vi "Parse Passport String.vi"(11 "Passport String":string) -> (0 "Why Bad":T1, 1 "Valid?":bool, 3 "Passport Info":T2)   [LabVIEW 2020]
uses:
  Typedefs/Passport.ctl
  Typedefs/ecl.ctl
  <vilib>/Utility/Data Type/NI_Data Type.lvlib
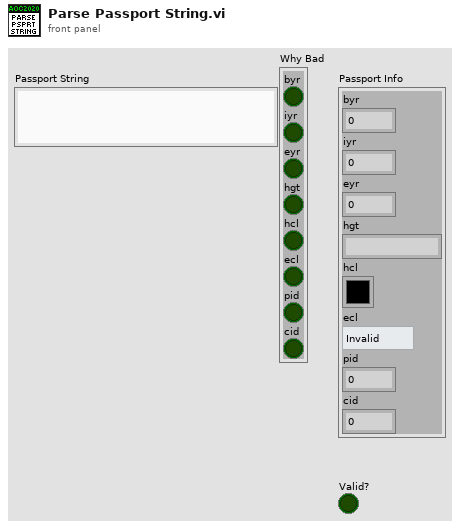
[diagram p1: front panel]
types:
  T1 = cluster{"byr":bool, "iyr":bool, "eyr":bool, "hgt":bool, "hcl":bool, "ecl":bool, "pid":bool, "cid":bool}
  T2 = typedef "Passport.ctl" = cluster{"byr":i32, "iyr":i32, "eyr":i32, "hgt":string, "hcl":u32, "ecl":T3, "pid":i32, "cid":i32}
  T3 = typedef "ecl.ctl" = enum16{"Invalid", "amb", "blu", "brn", "gry", "grn", "hzl", "oth"}
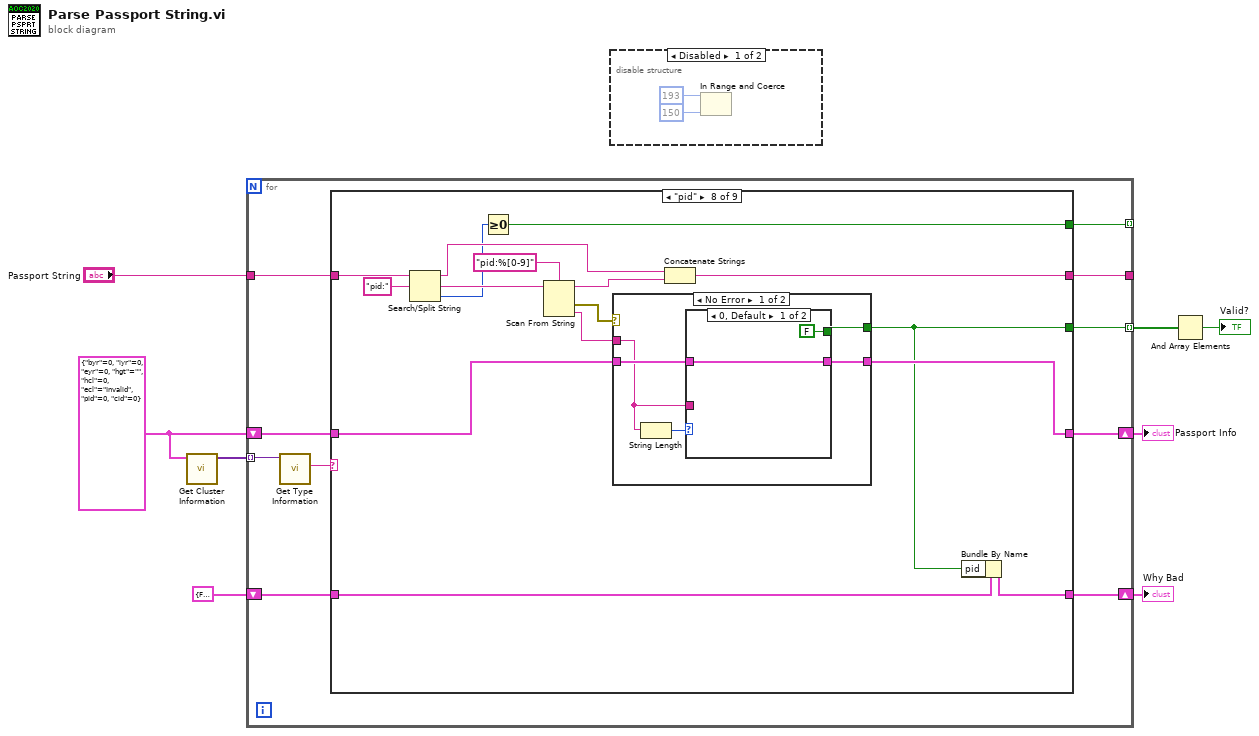
[diagram p0: block diagram]
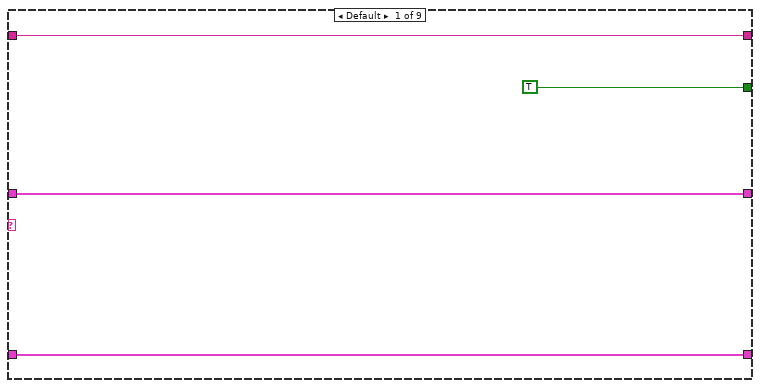
[diagram p3: hidden frame]
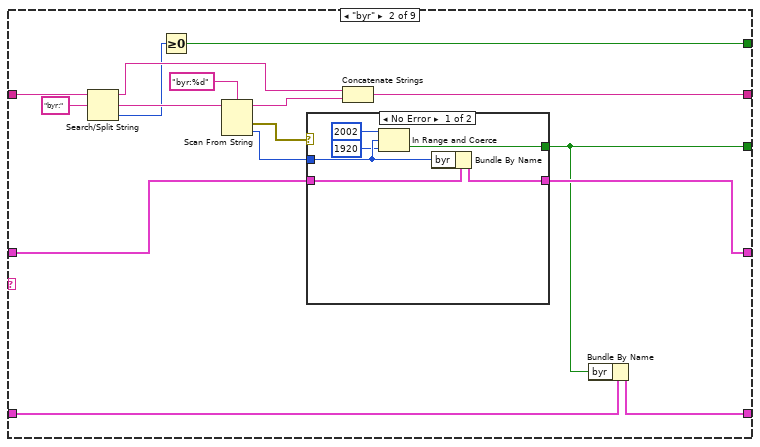
[diagram p4: hidden frame]
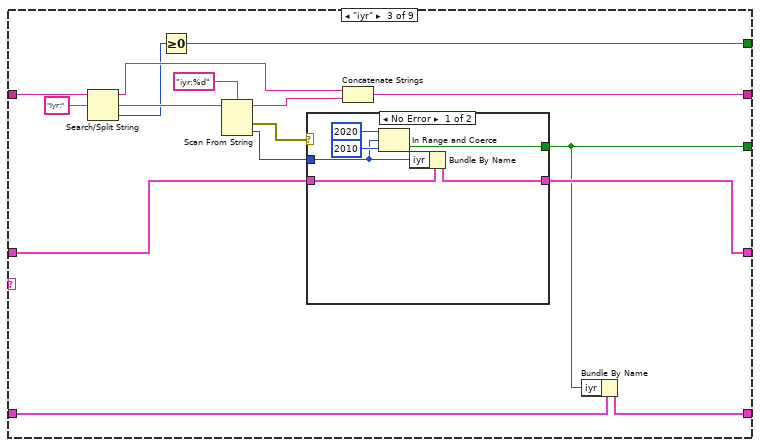
[diagram p6: hidden frame]
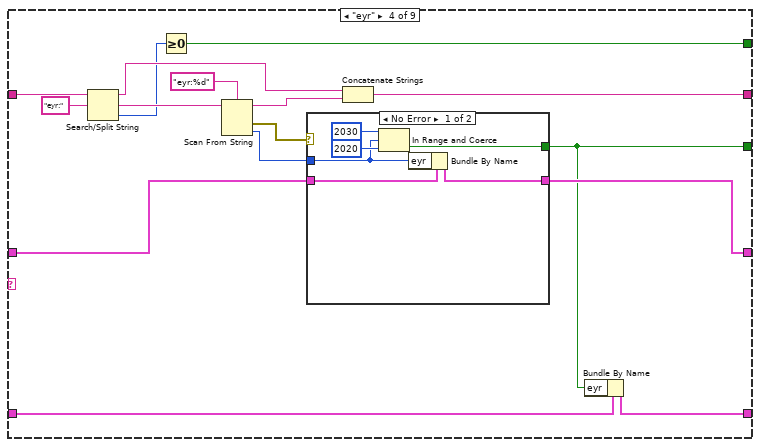
[diagram p8: hidden frame]
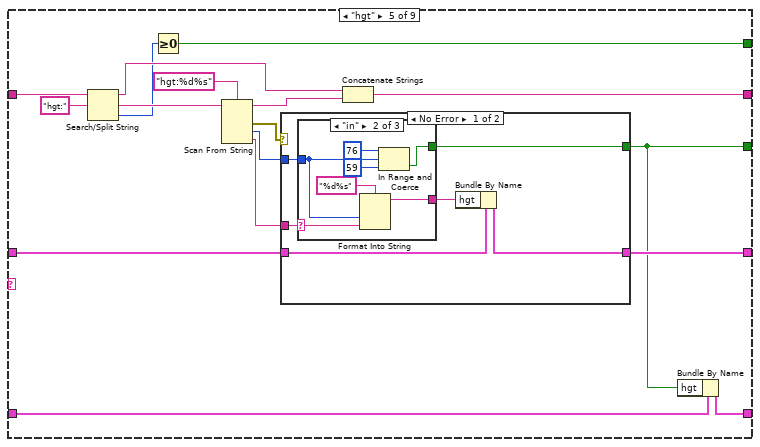
[diagram p10: hidden frame]
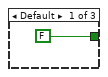
[diagram p11: hidden frame]
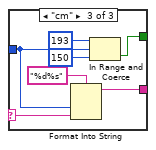
[diagram p12: hidden frame]
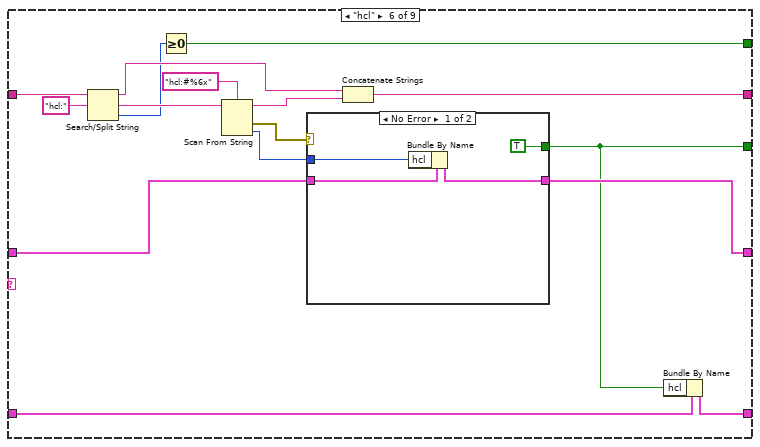
[diagram p14: hidden frame]
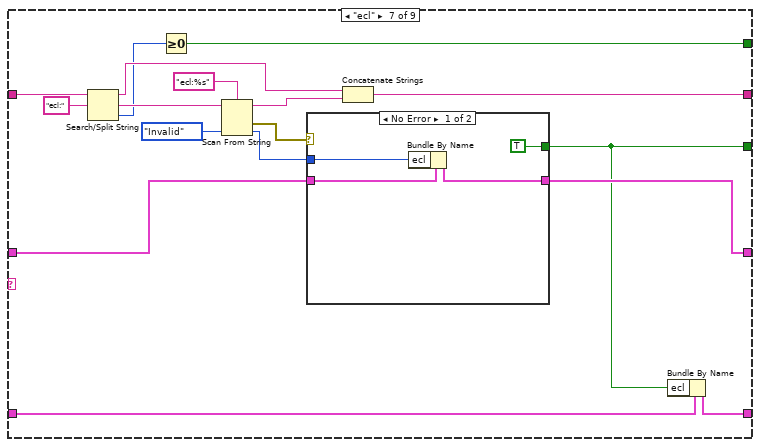
[diagram p16: hidden frame]
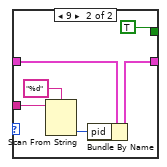
[diagram p18: hidden frame]
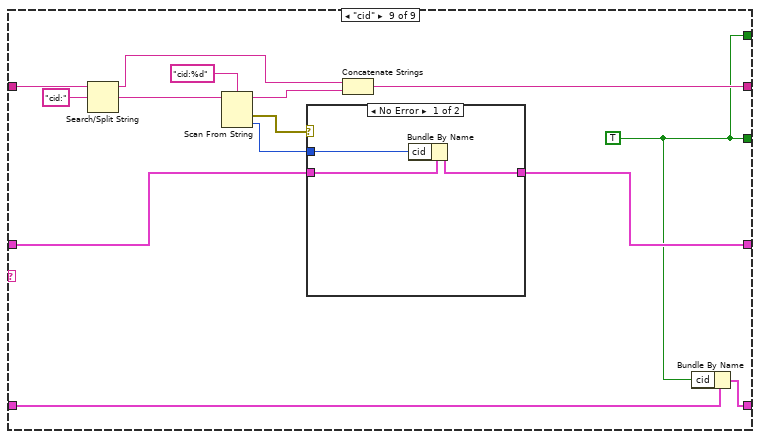
[diagram p20: hidden frame]
diagram:
  w3 = T2 {"byr"=0, "iyr"=0, "eyr"=0, "hgt"="", "hcl"=0, "ecl"=enum."Invalid", "pid"=0, "cid"=0}
  n1 = call <vilib>:"Get Cluster Information.vi"("variant"=w3) -> ("cluster elements"=w8:variant[])  [unwired: 9 in, 1 out]
  n2 = for {
    tunnel: w8 -> [w18] mode=indexing
    shift-right: [w15] -> w7
    shift-left: w3 -> [w14]
    tunnel: [w12] -> w4 mode=indexing
    tunnel: "Passport String" -> [w16]
    tunnel: [w13] -> _
    tunnel: [w11] -> _ mode=indexing
    shift-right: [w9] -> w1
    shift-left: T1 {"byr"=FALSE, "iyr"=FALSE, "eyr"=FALSE, "hgt"=FALSE, "hcl"=FALSE, "ecl"=FALSE, "pid"=FALSE, "cid"=FALSE} ("x = y?") -> [w10]
    n3 = call <vilib>:"Get Type Information.vi"("variant"=w18) -> ("name"=w17:string)  [unwired: 6 in, 4 out]
    n4 = case shown="\"pid\"" w17 {
      tunnel: w16 -> [w21 w34 w57 w80 w104 w142 w164 w185 w213]
      tunnel: [w22 w35 w58 w81 w105 w143 w165 w186 w214] -> w15
      tunnel: w14 -> [w22 w36 w59 w82 w106 w144 w166 w187 w215]
      tunnel: [w21 w29 w52 w75 w99 w137 w159 w180 w208] -> w13
      tunnel: [TRUE w23 w46 w69 w92 w131 w152 w174 w204] -> w12
      tunnel: [_ w26 w49 w72 w96 w134 w156 w177 w204] -> w11
      tunnel: w10 -> [w19 w25 w48 w71 w94 w132 w153 w175 w205]
      tunnel: [w19 w24 w47 w70 w93 w133 w154 w176 w206] -> w9
      frame Default {
      }
      frame "byr" {
        n5 = Search/Split String(string=w34, search string/char (-)="byr:" ("format string")) -> (substring before match=w30:string, match + rest of string=w32:string, offset of match=w27:i32)  [unwired: 1 in]
        n6 = Greater Or Equal To 0?(x=w27) -> (x >= 0?=w26:bool)
        n7 = Scan From String(format string="byr:%d", input string=w32) -> (remaining string=w31:string, error out=w37:errorcluster, output 1=w28:i32)  [unwired: 3 in, 1 out]
        n8 = case shown="No Error" w37 {
          tunnel: w36 -> [w44 w45]
          tunnel: [w43 w45] -> w35
          tunnel: w28 -> [w42 _]
          tunnel: [w41 _] -> w23
          frame No Error {
            n9 = In Range and Coerce(upper limit=2002, x=w42, lower limit=1920) -> (In Range?=w41:bool)  [unwired: 1 out]
            n10 = Bundle By Name(cluster=w44, "byr"=w42) -> (w43:T2)
          }
          frame Error {
          }
        }
        n11 = Concatenate Strings(w30, w31) -> (w29:string)
        n12 = Bundle By Name(cluster=w25, "byr"=w23) -> (w24:T1)
      }
      frame "iyr" {
        n13 = Search/Split String(string=w57, search string/char (-)="iyr:" ("format string")) -> (substring before match=w53:string, match + rest of string=w55:string, offset of match=w50:i32)  [unwired: 1 in]
        n14 = Greater Or Equal To 0?(x=w50) -> (x >= 0?=w49:bool)
        n15 = Scan From String(format string="iyr:%d", input string=w55) -> (remaining string=w54:string, error out=w60:errorcluster, output 1=w51:i32)  [unwired: 3 in, 1 out]
        n16 = case shown="No Error" w60 {
          tunnel: w59 -> [w67 w68]
          tunnel: [w66 w68] -> w58
          tunnel: w51 -> [w63 _]
          tunnel: [w62 _] -> w46
          frame No Error {
            n17 = In Range and Coerce(upper limit=2020, x=w63, lower limit=2010) -> (In Range?=w62:bool)  [unwired: 1 out]
            n18 = Bundle By Name(cluster=w67, "iyr"=w63) -> (w66:T2)
          }
          frame Error {
          }
        }
        n19 = Concatenate Strings(w53, w54) -> (w52:string)
        n20 = Bundle By Name(cluster=w48, "iyr"=w46) -> (w47:T1)
      }
      frame "eyr" {
        n21 = Search/Split String(string=w80, search string/char (-)="eyr:" ("format string")) -> (substring before match=w76:string, match + rest of string=w78:string, offset of match=w73:i32)  [unwired: 1 in]
        n22 = Greater Or Equal To 0?(x=w73) -> (x >= 0?=w72:bool)
        n23 = Scan From String(format string="eyr:%d", input string=w78) -> (remaining string=w77:string, error out=w83:errorcluster, output 1=w74:i32)  [unwired: 3 in, 1 out]
        n24 = case shown="No Error" w83 {
          tunnel: w82 -> [w90 w91]
          tunnel: [w89 w91] -> w81
          tunnel: w74 -> [w86 _]
          tunnel: [w85 _] -> w69
          frame No Error {
            n25 = In Range and Coerce(upper limit=2030, x=w86, lower limit=2020) -> (In Range?=w85:bool)  [unwired: 1 out]
            n26 = Bundle By Name(cluster=w90, "eyr"=w86) -> (w89:T2)
          }
          frame Error {
          }
        }
        n27 = Concatenate Strings(w76, w77) -> (w75:string)
        n28 = Bundle By Name(cluster=w71, "eyr"=w69) -> (w70:T1)
      }
      frame "hgt" {
        n29 = Search/Split String(string=w104, search string/char (-)="hgt:" ("format string")) -> (substring before match=w100:string, match + rest of string=w102:string, offset of match=w97:i32)  [unwired: 1 in]
        n30 = Greater Or Equal To 0?(x=w97) -> (x >= 0?=w96:bool)
        n31 = Scan From String(format string="hgt:%d%s", input string=w102) -> (remaining string=w101:string, error out=w107:errorcluster, output 1=w98:i32, output 2=w95:string)  [unwired: 4 in, 1 out]
        n32 = case shown="No Error" w107 {
          tunnel: w106 -> [w114 w130]
          tunnel: [w113 w130] -> w105
          tunnel: w98 -> [w111 _]
          tunnel: [w110 _] -> w92
          tunnel: w95 -> [w112 _]
          frame No Error {
            n33 = case shown="\"in\"" w112 {
              selector: w112 -> [_ w118 w125]
              tunnel: w111 -> [_ w117 w124]
              tunnel: [FALSE w120 w127] -> w110
              tunnel: [_ w116 w123] -> w109
              frame Default {
              }
              frame "in" {
                n34 = Format Into String(format string="%d%s", w117, w118) -> (resulting string=w116:string)  [unwired: 2 in, 1 out]
                n35 = In Range and Coerce(upper limit=76, x=w117, lower limit=59) -> (In Range?=w120:bool)  [unwired: 1 out]
              }
              frame "cm" {
                n36 = Format Into String(format string="%d%s", w124, w125) -> (resulting string=w123:string)  [unwired: 2 in, 1 out]
                n37 = In Range and Coerce(upper limit=193, x=w124, lower limit=150) -> (In Range?=w127:bool)  [unwired: 1 out]
              }
            }
            n38 = Bundle By Name(cluster=w114, "hgt"=w109) -> (w113:T2)
          }
          frame Error {
          }
        }
        n39 = Concatenate Strings(w100, w101) -> (w99:string)
        n40 = Bundle By Name(cluster=w94, "hgt"=w92) -> (w93:T1)
      }
      frame "hcl" {
        n41 = Search/Split String(string=w142, search string/char (-)="hcl:" ("format string")) -> (substring before match=w138:string, match + rest of string=w140:string, offset of match=w135:i32)  [unwired: 1 in]
        n42 = Greater Or Equal To 0?(x=w135) -> (x >= 0?=w134:bool)
        n43 = Scan From String(format string="hcl:#%6x", input string=w140) -> (remaining string=w139:string, error out=w145:errorcluster, output 1=w136:u32)  [unwired: 3 in, 1 out]
        n44 = case shown="No Error" w145 {
          tunnel: w144 -> [w150 w151]
          tunnel: [w149 w151] -> w143
          tunnel: w136 -> [w148 _]
          tunnel: [TRUE _] -> w131
          frame No Error {
            n45 = Bundle By Name(cluster=w150, "hcl"=w148) -> (w149:T2)
          }
          frame Error {
          }
        }
        n46 = Concatenate Strings(w138, w139) -> (w137:string)
        n47 = Bundle By Name(cluster=w132, "hcl"=w131) -> (w133:T1)
      }
      frame "ecl" {
        n48 = Search/Split String(string=w164, search string/char (-)="ecl:" ("format string")) -> (substring before match=w160:string, match + rest of string=w162:string, offset of match=w157:i32)  [unwired: 1 in]
        n49 = Greater Or Equal To 0?(x=w157) -> (x >= 0?=w156:bool)
        n50 = Scan From String(format string="ecl:%s", input string=w162, default 1=ecl."Invalid" ("ecl")) -> (remaining string=w161:string, error out=w167:errorcluster, output 1=w158:T3)  [unwired: 2 in, 1 out]
        n51 = case shown="No Error" w167 {
          tunnel: w166 -> [w172 w173]
          tunnel: [w171 w173] -> w165
          tunnel: w158 -> [w170 _]
          tunnel: [TRUE _] -> w152
          frame No Error {
            n52 = Bundle By Name(cluster=w172, "ecl"=w170) -> (w171:T2)
          }
          frame Error {
          }
        }
        n53 = Concatenate Strings(w160, w161) -> (w159:string)
        n54 = Bundle By Name(cluster=w153, "ecl"=w152) -> (w154:T1)
      }
      frame "pid" {
        n55 = Search/Split String(string=w185, search string/char (-)="pid:" ("format string")) -> (substring before match=w181:string, match + rest of string=w183:string, offset of match=w178:i32)  [unwired: 1 in]
        n56 = Greater Or Equal To 0?(x=w178) -> (x >= 0?=w177:bool)
        n57 = Scan From String(format string="pid:%[0-9]", input string=w183) -> (remaining string=w182:string, error out=w188:errorcluster, output 1=w179:string)  [unwired: 3 in, 1 out]
        n58 = case shown="No Error" w188 {
          tunnel: w187 -> [w194 w203]
          tunnel: [w193 w203] -> w186
          tunnel: w179 -> [w191 _]
          tunnel: [w192 _] -> w174
          frame No Error {
            n59 = String Length(string=w191) -> (length=w190:i32)
            n60 = case shown="0, Default" w190 {
              tunnel: w194 -> [w195 w202]
              tunnel: [w195 w201] -> w193
              tunnel: [FALSE TRUE] -> w192
              tunnel: w191 -> [_ w199]
              frame 0, Default {
              }
              frame 9 {
                n61 = Scan From String(format string="%d", input string=w199) -> (output 1=w197:i32)  [unwired: 3 in, 3 out]
                n62 = Bundle By Name(cluster=w202, "pid"=w197) -> (w201:T2)
              }
            }
          }
          frame Error {
          }
        }
        n63 = Concatenate Strings(w181, w182) -> (w180:string)
        n64 = Bundle By Name(cluster=w175, "pid"=w174) -> (w176:T1)
      }
      frame "cid" {
        w204 = TRUE
        n65 = Search/Split String(string=w213, search string/char (-)="cid:" ("format string")) -> (substring before match=w209:string, match + rest of string=w211:string)  [unwired: 1 in, 1 out]
        n66 = Scan From String(format string="cid:%d", input string=w211) -> (remaining string=w210:string, error out=w216:errorcluster, output 1=w207:i32)  [unwired: 3 in, 1 out]
        n67 = case shown="No Error" w216 {
          tunnel: w215 -> [w220 w221]
          tunnel: [w219 w221] -> w214
          tunnel: w207 -> [w218 _]
          frame No Error {
            n68 = Bundle By Name(cluster=w220, "cid"=w218) -> (w219:T2)
          }
          frame Error {
          }
        }
        n69 = Concatenate Strings(w209, w210) -> (w208:string)
        n70 = Bundle By Name(cluster=w205, "cid"=w204) -> (w206:T1)
      }
    }
  }
  "Passport Info" <- w7
  "Why Bad" <- w1
  n71 = disable-structure shown="Disabled" {
    frame Disabled {
      n72 = In Range and Coerce(upper limit=193, lower limit=150) -> ()  [unwired: 1 in, 2 out]
    }
    frame Enabled {
    }
  }
  n73 = And Array Elements(Boolean array=w4) -> (logical AND=→"Valid?":bool)
